vi "T11.vi"(2 "Parametry Ziemi":T1={"a - półoś duża"=6378137.0, "b - półoś mała"=6356752.3141999999998} {"b - półoś mała" format="%_20f"; "a - półoś duża" format="%_20g"}, 3 "fi'":ext) -> (7 "T11":ext)   [LabVIEW 2015, in "Biblioteka moduł map v3.lvlib" / "Konwersja wsp.lvlib" / "UTM.lvlib" / "Konwersja z UTM na wsp geograficzne.lvlib"]
uses:
  Konwersja z UTM na wsp geograficzne.lvlib
  UTM.lvlib
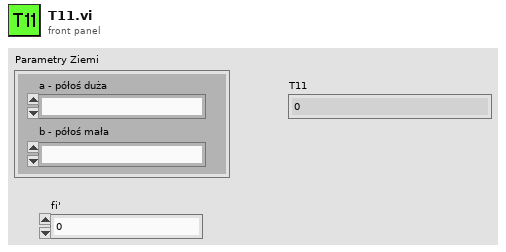
[diagram p1: front panel]
types:
  T1 = cluster{"a - półoś duża":ext, "b - półoś mała":ext}
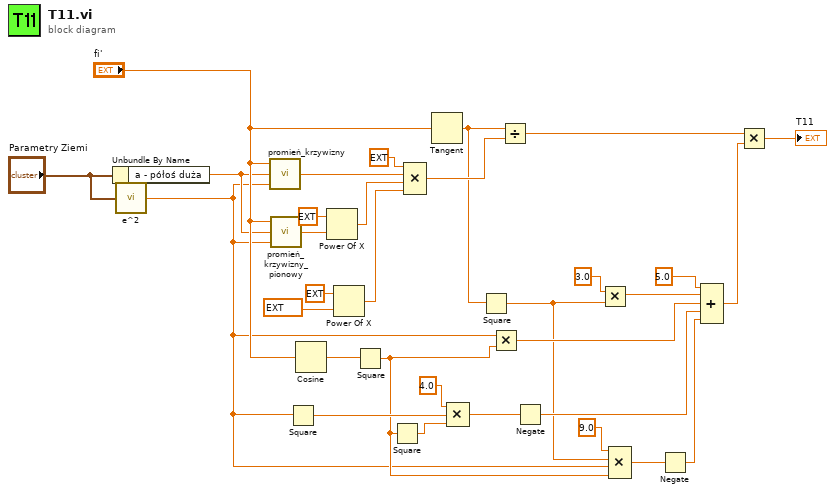
[diagram p0: block diagram]
diagram:
  n1 = Unbundle By Name("Parametry Ziemi") -> ("a - półoś duża"=w3:ext)
  n2 = call "e^2.vi"("Parametry Ziemi"="Parametry Ziemi") -> ("e^2"=w2:ext)  [unwired: 4 in]
  n3 = call "promień_krzywizny.vi"("e^2"=w2, "a"=w3, "fi[rad]"="fi'") -> ("Promien krzywizny południka"=w30:ext)  [unwired: 2 in]
  n4 = call "promień_krzywizny_pionowy.vi"("e^2"=w2, "a"=w3, "fi[rad]"="fi'") -> ("Promien krzywizny równoleżnika"=w29:ext)  [unwired: 2 in]
  n5 = Square(x=w2) -> (x^2=w10:ext)
  n6 = Cosine(x="fi'") -> (cos(x)=w15:ext)
  n7 = Power Of X(1:w29, 2:ext 3.0 ("y")) -> (0:w25:ext)
  n8 = Power Of X(1:ext 0.9996 ("k0"), 2:ext 4.0 ("y")) -> (0:w24:ext)
  n9 = Square(x=w15) -> (x^2=w4:ext)
  n10 = Square(x=w4) -> (x^2=w9:ext)
  n11 = Compound Arithmetic op=MULTIPLY(ext 24.0 ("value"), w30, w25, w24) -> (w32:ext)
  n12 = Tangent(1:"fi'") -> (0:w17:ext)
  n13 = Compound Arithmetic op=MULTIPLY(4.0 ("value"), w10, w9) -> (w13:ext)
  n14 = Square(x=w17) -> (x^2=w5:ext)
  n15 = Multiply(x=w2, y=w4) -> (x*y=w16:ext)
  n16 = Divide(x=w17, y=w32) -> (x/y=w23:ext)
  n17 = Negate(x=w13) -> (-x=w12:ext)
  n18 = Multiply(x=3.0, y=w5) -> (x*y=w19:ext)
  n19 = Compound Arithmetic op=MULTIPLY(9.0 ("value"), w5, w2, w4) -> (w8:ext)
  n20 = Negate(x=w8) -> (-x=w7:ext)
  n21 = Compound Arithmetic op=ADD(5.0 ("value"), w19, w16, w12, w7) -> (w21:ext)
  n22 = Multiply(x=w23, y=w21) -> (x*y=→"T11":ext)
